vi "Read daemon error.vi"(8 "error in (no error)":errorcluster, 11 "network slave in":refnum<class "Network Slave.lvclass">) -> (0 "error out":errorcluster, 2 "daemon error":errorcluster, 3 "network slave out":refnum<class "Network Slave.lvclass">)   [LabVIEW 2017, in "SubVIs.lvlib" / "Network Slave.lvclass"]
uses:
  <vilib>/Modbus/subvis/Protocol/Interfaces/Network Slave/Network Slave.lvclass
  <vilib>/Modbus/subvis/Protocol/Interfaces/Network Slave/Network Slave.lvclass/Network Slave.ctl
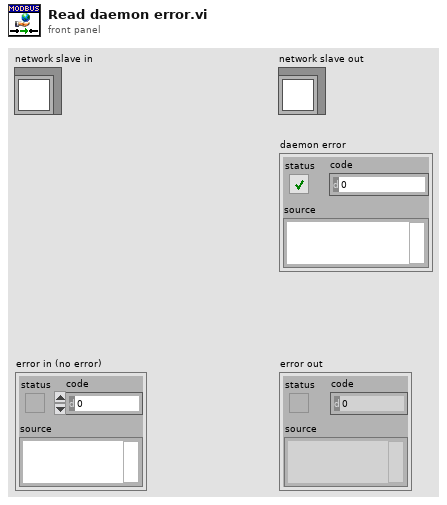
[diagram p1: front panel]
types:
  T1 = typedef "SubVIs.lvlib/Network Slave.lvclass/daemon status cluster.ctl" = cluster{"error":errorcluster, "status":enum16{"Not Started", "Running", "Error", "Stopped"}}
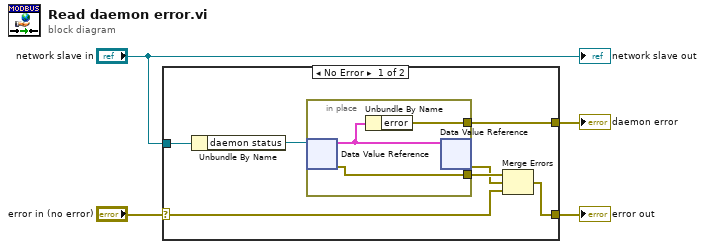
[diagram p0: block diagram]
diagram:
  n1 = case shown="No Error" "error in (no error)" {
    selector: "error in (no error)" -> [w5 w15]
    tunnel: [w10 w15] -> w4
    tunnel: "network slave in" -> [w9 _]
    tunnel: [w8 _] -> w2
    frame No Error {
      n2 = Unbundle By Name(w9) -> ("daemon status"=w11:refnum<data-value>)
      n3 = in-place {
        in-place-border: [w13] -> w8
        in-place-border: [w12] -> w7
        n4 = in-place-dvr #1(w11) -> (w14:T1, w12:errorcluster)
        n5 = Unbundle By Name(w14) -> ("error"=w13:errorcluster)
        n6 = in-place-dvr #1(w14) -> (w6:errorcluster)  [unwired: 1 out]
      }
      n7 = Merge Errors(w7, w6, w5) -> (w10:errorcluster)
    }
    frame Error {
    }
  }
  "error out" <- w4
  "daemon error" <- w2
  "network slave out" <- "network slave in"
